vi "TEST_02_ui_plot_window.vi"() -> ()   [LabVIEW 2025]
uses:
  166e0385-1291-4ee6-a608-8b02bdaae3d2.vi
  b1158e5f-e22e-42fa-9d41-9ea4e4d0b9e3.vi
  9c1d92a2-1c85-4809-97a6-d36bf52cbad7.vi
  d684625a-03c4-4daf-8e9e-674a236ebb3e.vi
  fb960f78-e1fe-4b5d-8417-6d8be925c5cf.vi
  c135c75a-78bf-4448-8d92-d4bbbd51cd11.vi
  00_global_variables.vi
panel:
  out "plot_0":cluster{"array type (2D Dbl)":dbl[], dbl[]}[](graph)
  in  "select_plot_3":string(combo)="2"
  in  "select_plot_2":string(combo)="2"
  in  "select_plot_1":string(combo)="2"
  in  "select_plot_0":string(combo)="2"
  out "cursor_p3_1_prefix":string
  out "cursor_p2_1_prefix":string
  out "cursor_p1_1_prefix":string
  out "cursor_p0_1_prefix":string
  out "cursor_p3_2_prefix":string
  out "cursor_p2_2_prefix":string
  out "cursor_p1_2_prefix":string
  out "cursor_p0_2_prefix":string
  out "cursor_p3_2":dbl format="%#_6f"
  in  "color_picker_3":u32(colorbox)=14468608
  out "cursor_p3_1":dbl format="%#_6f"
  in  "enable_plot_3":bool=TRUE caption="S11 - Imaginary"
  out "cursor_p2_2":dbl format="%#_6f"
  in  "color_picker_2":u32(colorbox)=39219
  out "cursor_p2_1":dbl format="%#_6f"
  in  "enable_plot_2":bool caption="S11 - Imaginary"
  out "cursor_p1_2":dbl format="%#_6f"
  out "cursor_p0_2":dbl format="%#_6f"
  out "cursor_p0_freq_2":string caption="Frequenz"
  out "cursor_p0_wavel_2":dbl caption="Frequenz"
  out "cursor_p0_wavel_1":dbl caption="Frequenz"
  in  "color_picker_1":u32(colorbox)=14423100
  in  "color_picker_0":u32(colorbox)=26316
  out "cursor_p0_freq_1":string caption="Frequenz"
  out "cursor_p1_1":dbl format="%#_6f"
  out "cursor_p0_1":dbl format="%#_6f"
  in  "enable_plot_1":bool caption="S11 - Imaginary"
  in  "enable_plot_0":bool=TRUE
  # "Hz"
  # "Frequency"
  # "Hz"
  # "Wavelength"
  # "m"
  # "m"
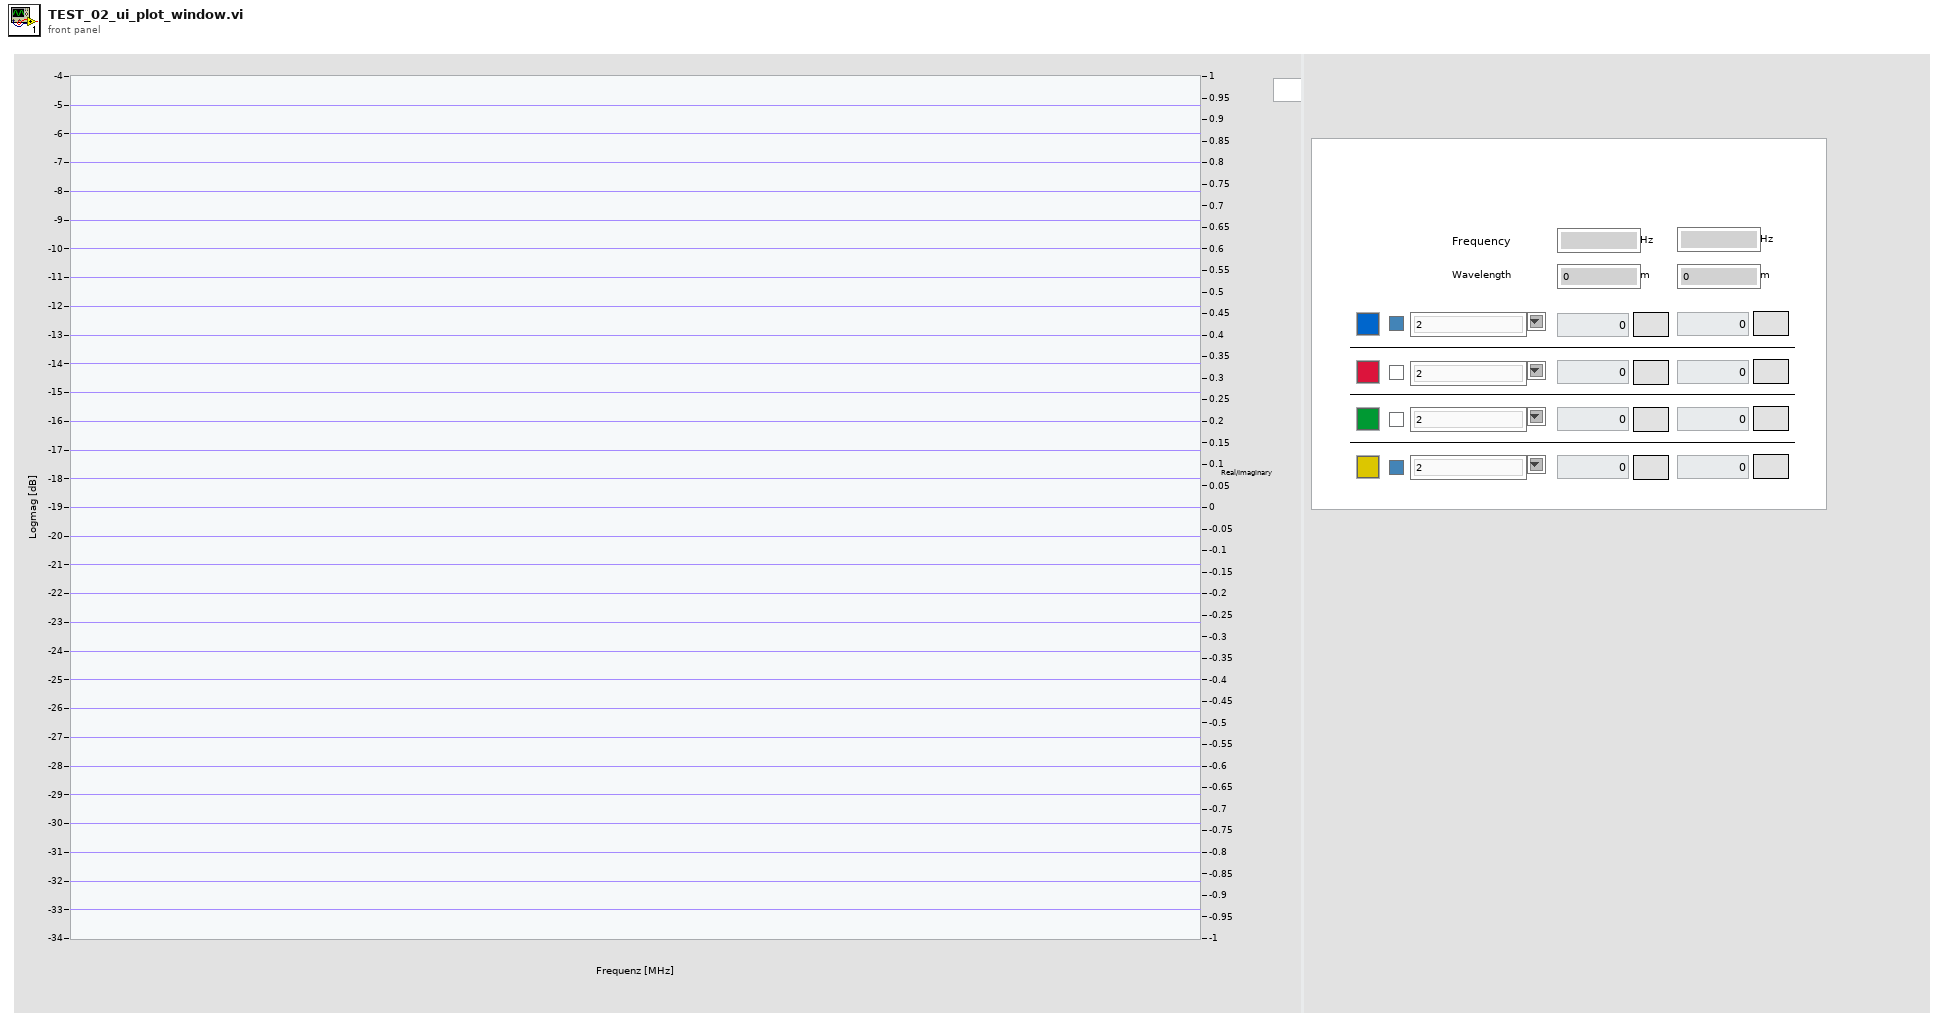
[diagram p1: front panel]
types:
  T1 = typedef "LVCursorListTypeDef.ctl" = cluster{"Name":string, "Color":u32, "Style":u8, "Point Style":u8, "Name Visible":bool, "Allow Drag":bool, "Cursor Mode":u32, "Plot":i32, "Index":i32, "Position":cluster{"X":dbl, "Y":dbl}, "X Scale":u32, "Y Scale":u32, "Watch Plots":i32[], "Watch All Plots":bool, "Plot Area":i32, "Label Offset":cluster{"X":dbl, "Y":dbl}}[]
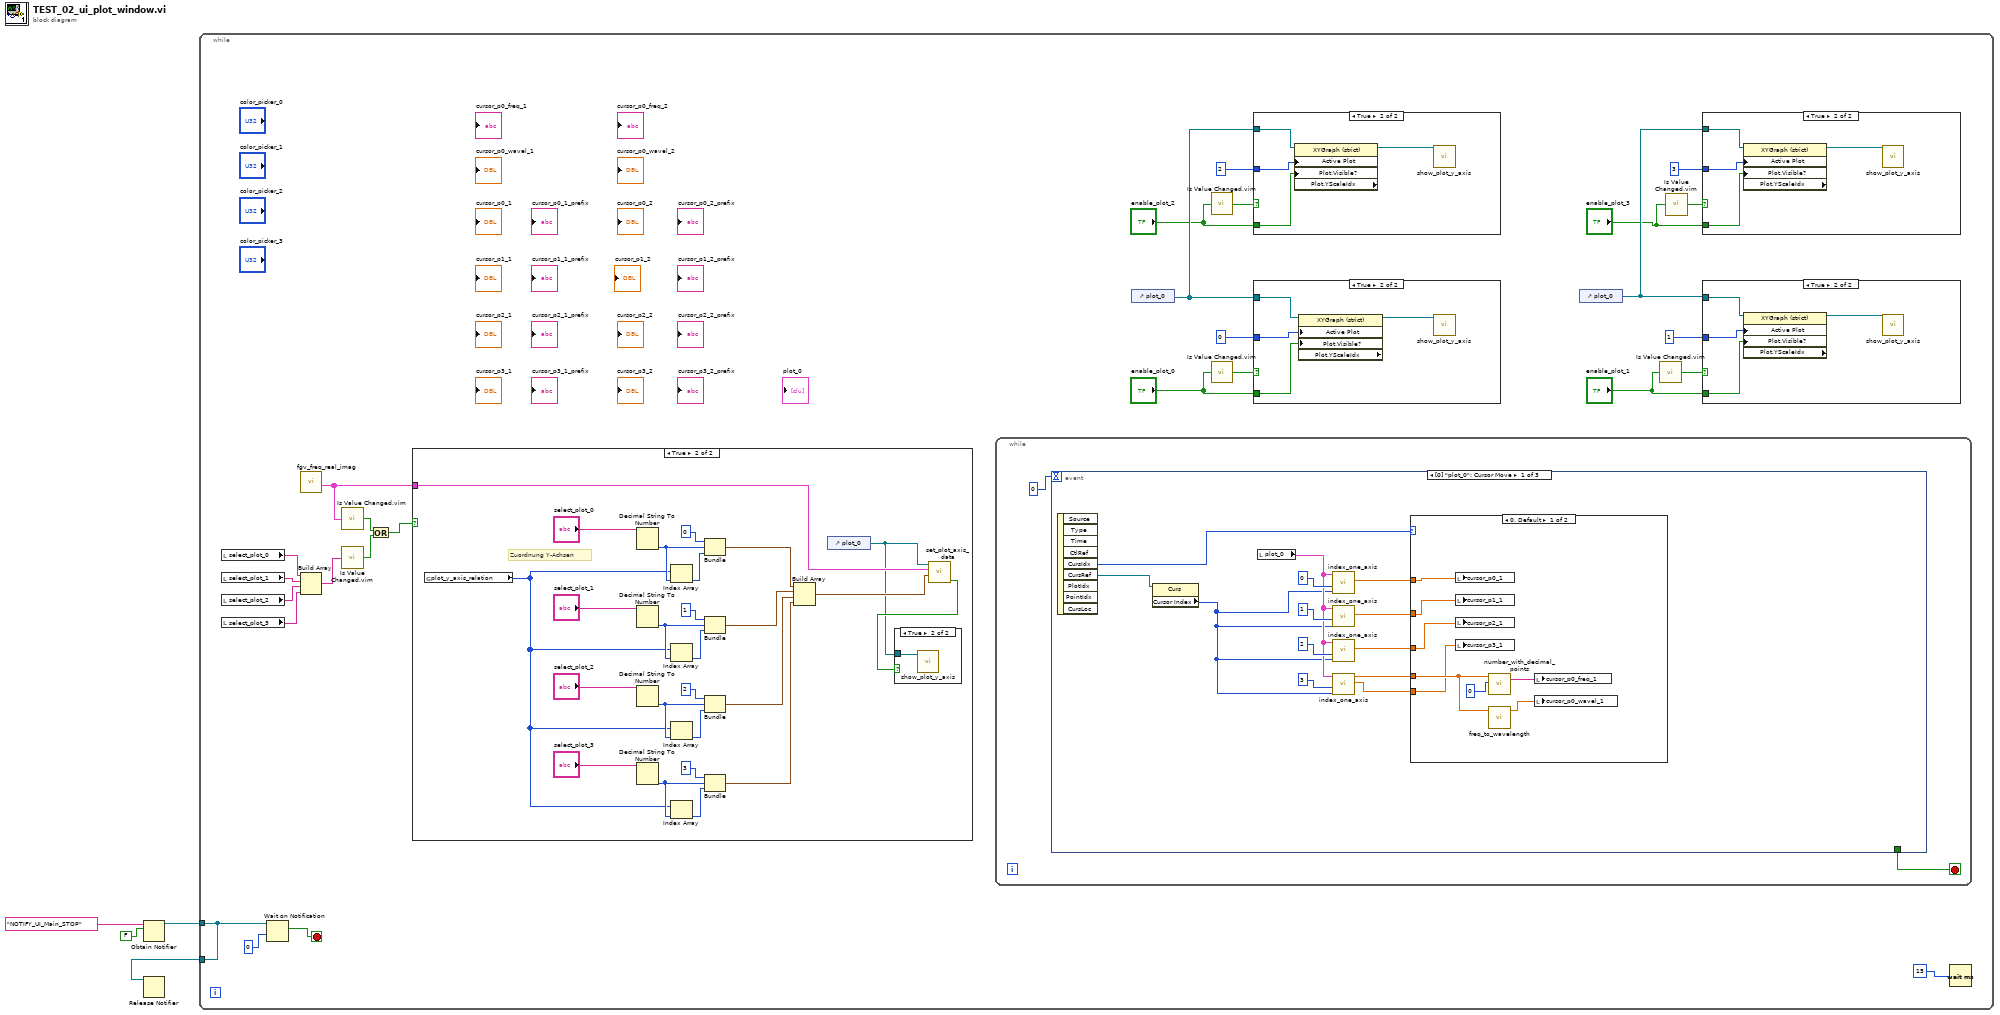
[diagram p0: block diagram]
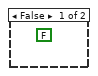
[diagram p3: hidden frame]
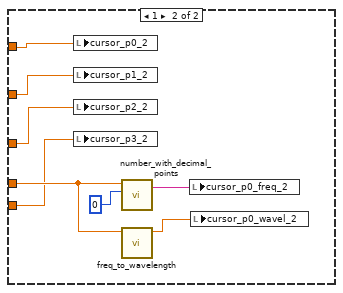
[diagram p8: hidden frame]
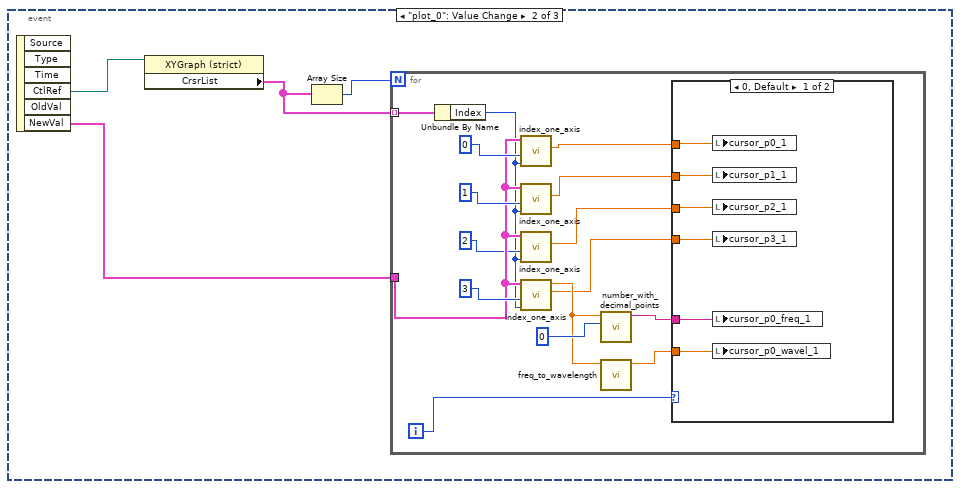
[diagram p9: hidden frame]
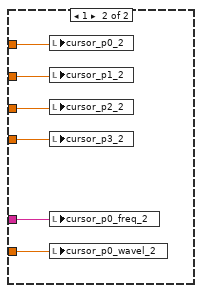
[diagram p10: hidden frame]
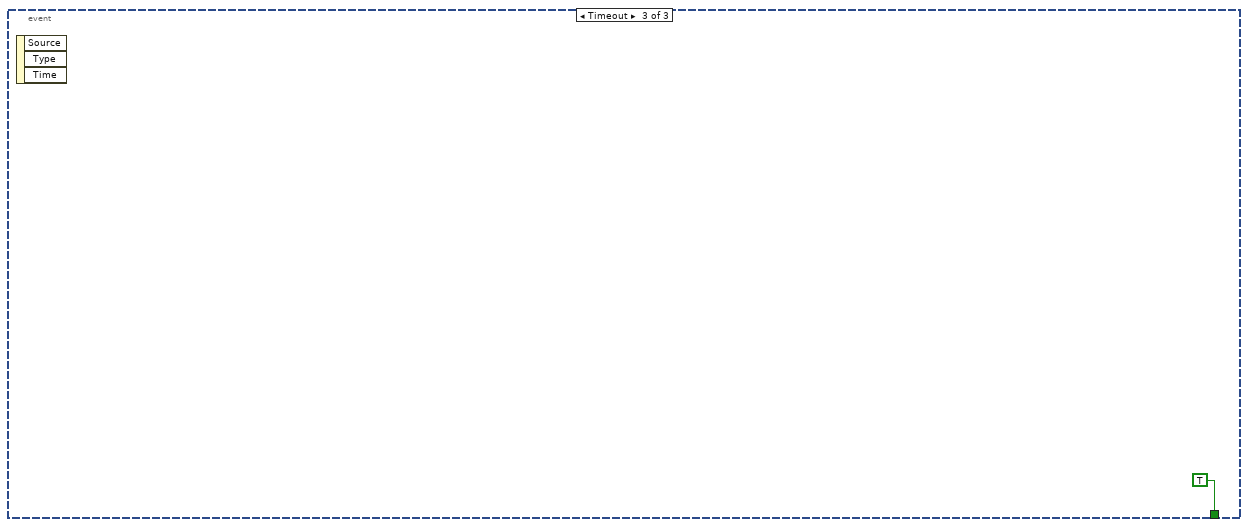
[diagram p11: hidden frame]
diagram:
  n1 = Obtain Notifier(name (unnamed)="NOTIFY_UI_Main_STOP", notification data type=FALSE) -> (notifier out=w2:refnum<notifier>)  [unwired: 2 in, 2 out]
  n2 = while {
    tunnel: w2 -> [w8]
    tunnel: [w8] -> w1
    stop <- w7 stop-if-true
    n3 = local read "select_plot_0"() -> (w20:string)
    n4 = local read "select_plot_1"() -> (w19:string)
    n5 = local read "select_plot_2"() -> (w18:string)
    n6 = local read "select_plot_3"() -> (w17:string)
    n7 = Wait on Notification(notifier=w8, timeout in ms (-1)=0) -> (notification=w7:bool)  [unwired: 2 in, 3 out]
    n8 = call "fgv_freq_real_imag.vi"() -> ("plot_data"=w5:cluster{"freq_array":dbl[], "X2":dbl[]}[])  [unwired: 8 in, 3 out]
    n9 = Build Array(w20, w19, w18, w17) -> (w16:string[])
    n10 = call "Is Value Changed.vim"("value"=w5) -> ("changed or first call?"=w21:bool)
    n11 = call "Is Value Changed.vim"("value"=w16) -> ("changed or first call?"=w15:bool)
    n12 = Or(x=w21, y=w15) -> (x .or. y?=w22:bool)
    n13 = case shown="True" w22 {
      tunnel: w5 -> [_ w39]
      frame False {
        (unwired) FALSE
      }
      frame True {
        # "Zuordnung Y-Achsen"
        n14 = global read "00_global_variables.vi" "plot_y_axis_relation"() -> (w36:i32[])
        n15 = Decimal String To Number(string="select_plot_0") -> (number=w48:i32)  [unwired: 2 in, 1 out]
        n16 = Decimal String To Number(string="select_plot_1") -> (number=w46:i32)  [unwired: 2 in, 1 out]
        n17 = Decimal String To Number(string="select_plot_2") -> (number=w44:i32)  [unwired: 2 in, 1 out]
        n18 = Decimal String To Number(string="select_plot_3") -> (number=w42:i32)  [unwired: 2 in, 1 out]
        n19 = Index Array(array=w36, index=w48) -> (element=w47:i32)
        n20 = Index Array(array=w36, index=w46) -> (element=w45:i32)
        n21 = Index Array(array=w36, index=w44) -> (element=w43:i32)
        n22 = Index Array(array=w36, index=w42) -> (element=w41:i32)
        n23 = Bundle(0, w48, w47) -> (w57:cluster{i32, i32, i32})  [unwired: 1 in]
        n24 = Bundle(1, w46, w45) -> (w58:cluster{i32, i32, i32})  [unwired: 1 in]
        n25 = Bundle(2, w44, w43) -> (w59:cluster{i32, i32, i32})  [unwired: 1 in]
        n26 = Bundle(3, w42, w41) -> (w53:cluster{i32, i32, i32})  [unwired: 1 in]
        n27 = Build Array(w57, w58, w59, w53) -> (w40:cluster{i32, i32, i32}[])
        n28 = control-ref of="plot_0"() -> (w37:refnum<vi>)
        n29 = call "set_plot_axis_data.vi"("plot_allocation"=w40, "plot_data"=w39, "reference"=w37) -> ("done"=w38:bool)  [unwired: 8 in]
        n30 = case shown="True" w38 {
          tunnel: w37 -> [_ w61]
          frame False {
          }
          frame True {
            n31 = call "show_plot_y_axis.vi"("plot_ref"=w61) -> ()  [unwired: 10 in, 1 out]
          }
        }
      }
    }
    n32 = while {
      stop <- w75 stop-if-true
      n33 = event shown="[0] \"plot_0\": Cursor Move" {
        selector: _ -> [_ _ _]
        dyn-events: _ -> [_ _ _]
        timeout: 0 -> [_ _ _]
        tunnel: [_ _ TRUE] -> w75
        event "plot_0": Cursor Move {
          n34 = event-data() -> ("CursIdx"=w80:i32, "CursRef"=w81:refnum<vi>)  [unwired: 1 in, 7 out]
          n35 = property on="Property Node" class="Curs"(reference=w81) -> ("Cursor Index"=w76:i32)  [unwired: 1 in, 2 out]
          n36 = local read "plot_0"() -> (w78:cluster{"array type (2D Dbl)":dbl[], dbl[]}[])
          n37 = call "index_one_axis.vi"("x_index"=w76, "curve_sel"=0 ("x_index"), "graph_data"=w78) -> ("Y"=w88:dbl)  [unwired: 7 in, 1 out]
          n38 = call "index_one_axis.vi"("x_index"=w76, "curve_sel"=1 ("x_index"), "graph_data"=w78) -> ("Y"=w87:dbl)  [unwired: 7 in, 1 out]
          n39 = call "index_one_axis.vi"("x_index"=w76, "curve_sel"=2 ("x_index"), "graph_data"=w78) -> ("Y"=w77:dbl)  [unwired: 7 in, 1 out]
          n40 = call "index_one_axis.vi"("x_index"=w76, "curve_sel"=3 ("x_index"), "graph_data"=w78) -> ("Y"=w85:dbl, "X"=w86:dbl)  [unwired: 7 in]
          n41 = case shown="0, Default" w80 {
            tunnel: w85 -> [w89 w97]
            tunnel: w86 -> [w91 w101]
            tunnel: w87 -> [w92 w100]
            tunnel: w88 -> [w93 w99]
            tunnel: w77 -> [w90 w98]
            frame 0, Default {
              n42 = local write "cursor_p0_1"(w93) -> ()
              n43 = local write "cursor_p1_1"(w92) -> ()
              n44 = local write "cursor_p2_1"(w90) -> ()
              n45 = local write "cursor_p3_1"(w89) -> ()
              n46 = call "number_with_decimal_points.vi"("Precision"=i16 0, "Double"=w91) -> ("String"=w95:string)  [unwired: 5 in]
              n47 = call "freq_to_wavelength.vi"("frequency_hz"=w91) -> ("wavelength_m"=w94:dbl)  [unwired: 10 in]
              n48 = local write "cursor_p0_freq_1"(w95) -> ()
              n49 = local write "cursor_p0_wavel_1"(w94) -> ()
            }
            frame 1 {
              n50 = local write "cursor_p0_2"(w99) -> ()
              n51 = local write "cursor_p1_2"(w100) -> ()
              n52 = local write "cursor_p2_2"(w98) -> ()
              n53 = local write "cursor_p3_2"(w97) -> ()
              n54 = call "number_with_decimal_points.vi"("Precision"=i16 0, "Double"=w101) -> ("String"=w103:string)  [unwired: 5 in]
              n55 = call "freq_to_wavelength.vi"("frequency_hz"=w101) -> ("wavelength_m"=w102:dbl)  [unwired: 10 in]
              n56 = local write "cursor_p0_freq_2"(w103) -> ()
              n57 = local write "cursor_p0_wavel_2"(w102) -> ()
            }
          }
        }
        event "plot_0": Value Change {
          n58 = event-data() -> ("CtlRef"=w106:refnum<vi>, "NewVal"=w105:cluster{"array type (2D Dbl)":dbl[], dbl[]}[])  [unwired: 1 in, 4 out]
          n59 = property on="Property Node" class="XYGraph (strict)"(reference=w106) -> ("CrsrList"=w108:T1)  [unwired: 1 in, 2 out]
          n60 = Array Size(array=w108) -> (size(s)=w107:i32)
          n61 = for {
            N: w107 -> [_]
            tunnel: w108 -> [w124] mode=indexing
            tunnel: w105 -> [w113]
            i -> [w114]
            n62 = Unbundle By Name(w124) -> ("Index"=w111:i32)
            n63 = call "index_one_axis.vi"("x_index"=w111, "curve_sel"=0 ("x_index"), "graph_data"=w113) -> ("Y"=w117:dbl)  [unwired: 7 in, 1 out]
            n64 = call "index_one_axis.vi"("x_index"=w111, "curve_sel"=1 ("x_index"), "graph_data"=w113) -> ("Y"=w118:dbl)  [unwired: 7 in, 1 out]
            n65 = call "index_one_axis.vi"("x_index"=w111, "curve_sel"=2 ("x_index"), "graph_data"=w113) -> ("Y"=w110:dbl)  [unwired: 7 in, 1 out]
            n66 = call "index_one_axis.vi"("x_index"=w111, "curve_sel"=3 ("x_index"), "graph_data"=w113) -> ("Y"=w109:dbl, "X"=w116:dbl)  [unwired: 7 in]
            n67 = call "number_with_decimal_points.vi"("Precision"=i16 0, "Double"=w116) -> ("String"=w123:string)  [unwired: 5 in]
            n68 = call "freq_to_wavelength.vi"("frequency_hz"=w116) -> ("wavelength_m"=w115:dbl)  [unwired: 10 in]
            n69 = case shown="0, Default" w114 {
              tunnel: w123 -> [w130 w132]
              tunnel: w118 -> [w129 w135]
              tunnel: w117 -> [w128 w136]
              tunnel: w110 -> [w127 w134]
              tunnel: w115 -> [w126 w131]
              tunnel: w109 -> [w125 w133]
              frame 0, Default {
                n70 = local write "cursor_p0_1"(w128) -> ()
                n71 = local write "cursor_p1_1"(w129) -> ()
                n72 = local write "cursor_p2_1"(w127) -> ()
                n73 = local write "cursor_p3_1"(w125) -> ()
                n74 = local write "cursor_p0_freq_1"(w130) -> ()
                n75 = local write "cursor_p0_wavel_1"(w126) -> ()
              }
              frame 1 {
                n76 = local write "cursor_p0_2"(w136) -> ()
                n77 = local write "cursor_p1_2"(w135) -> ()
                n78 = local write "cursor_p2_2"(w134) -> ()
                n79 = local write "cursor_p3_2"(w133) -> ()
                n80 = local write "cursor_p0_freq_2"(w132) -> ()
                n81 = local write "cursor_p0_wavel_2"(w131) -> ()
              }
            }
          }
        }
        event Timeout {
          n82 = event-data() -> ()  [unwired: 1 in, 3 out]
        }
      }
    }
    n83 = control-ref of="plot_0"() -> (w24:refnum<vi>)
    n84 = call "Is Value Changed.vim"("value"="enable_plot_2") -> ("changed or first call?"=w26:bool)
    n85 = call "Is Value Changed.vim"("value"="enable_plot_0") -> ("changed or first call?"=w9:bool)
    n86 = case shown="True" w26 {
      tunnel: "enable_plot_2" -> [_ w62]
      tunnel: w24 -> [_ w65]
      tunnel: 2 ("plot_id") -> [_ w64]
      frame False {
      }
      frame True {
        n87 = property on="Property Node" class="XYGraph (strict)" props=["Active Plot", "Plot", "Visible?", "Plot", "YScaleIdx"](reference=w65, "Active Plot"=w64, "Plot.Visible?"=w62) -> (reference out=w63:refnum<vi>)  [unwired: 1 in, 2 out]
        n88 = call "show_plot_y_axis.vi"("plot_ref"=w63) -> ()  [unwired: 10 in, 1 out]
      }
    }
    n89 = case shown="True" w9 {
      tunnel: "enable_plot_0" -> [_ w71]
      tunnel: w24 -> [_ w73]
      tunnel: 0 ("plot_id") -> [_ w72]
      frame False {
      }
      frame True {
        n90 = property on="Property Node" class="XYGraph (strict)" props=["Active Plot", "Plot", "Visible?", "Plot", "YScaleIdx"](reference=w73, "Active Plot"=w72, "Plot.Visible?"=w71) -> (reference out=w70:refnum<vi>)  [unwired: 1 in, 2 out]
        n91 = call "show_plot_y_axis.vi"("plot_ref"=w70) -> ()  [unwired: 10 in, 1 out]
      }
    }
    n92 = control-ref of="plot_0"() -> (w14:refnum<vi>)
    n93 = call "Is Value Changed.vim"("value"="enable_plot_1") -> ("changed or first call?"=w29:bool)
    n94 = call "Is Value Changed.vim"("value"="enable_plot_3") -> ("changed or first call?"=w12:bool)
    n95 = case shown="True" w12 {
      tunnel: "enable_plot_3" -> [_ w32]
      tunnel: w14 -> [_ w35]
      tunnel: 3 ("plot_id") -> [_ w34]
      frame False {
      }
      frame True {
        n96 = property on="Property Node" class="XYGraph (strict)" props=["Active Plot", "Plot", "Visible?", "Plot", "YScaleIdx"](reference=w35, "Active Plot"=w34, "Plot.Visible?"=w32) -> (reference out=w33:refnum<vi>)  [unwired: 1 in, 2 out]
        n97 = call "show_plot_y_axis.vi"("plot_ref"=w33) -> ()  [unwired: 10 in, 1 out]
      }
    }
    n98 = case shown="True" w29 {
      tunnel: "enable_plot_1" -> [_ w66]
      tunnel: w14 -> [_ w69]
      tunnel: 1 ("plot_id") -> [_ w68]
      frame False {
      }
      frame True {
        n99 = property on="Property Node" class="XYGraph (strict)" props=["Active Plot", "Plot", "Visible?", "Plot", "YScaleIdx"](reference=w69, "Active Plot"=w68, "Plot.Visible?"=w66) -> (reference out=w67:refnum<vi>)  [unwired: 1 in, 2 out]
        n100 = call "show_plot_y_axis.vi"("plot_ref"=w67) -> ()  [unwired: 10 in, 1 out]
      }
    }
    n101 = Wait (ms)(milliseconds to wait=u32 15) -> ()  [unwired: 1 out]
  }
  n102 = Release Notifier(notifier=w1) -> ()  [unwired: 2 in, 3 out]
